vi "Update Sequence Params.vi"(8 "error in (no error)":errorcluster, 9 "Daq Channel Info In":T1, 10 "Sequence Parameters In":T2, 11 "UI in":refnum<class "UI.lvclass">) -> (0 "error out":errorcluster, 3 "UI out":refnum<class "UI.lvclass">)   [LabVIEW 2015, in "UI.lvlib" / "UI.lvclass"]
uses:
  UI.lvclass
  Sequencer/Sequencer/Sequence Parameters.ctl
  Sequencer/Sequencer/Daq Channel Info.ctl
  UI.lvclass/UI.ctl
  <vilib>/ActorFramework/Actor/Actor.lvclass/Actor.ctl
  <vilib>/ActorFramework/Message Enqueuer/Message Enqueuer.lvclass/Message Enqueuer.ctl
  <vilib>/ActorFramework/Message Enqueuer/Init from Existing Queue.vi
  <vilib>/ActorFramework/Message Enqueuer/Message Enqueuer.lvclass
  <vilib>/ActorFramework/Actor/Actor.lvclass
  UI Messages/Update Refs Msg/Update Refs Msg.lvclass
  Sequencer/Sequencer/Sequencer.lvclass
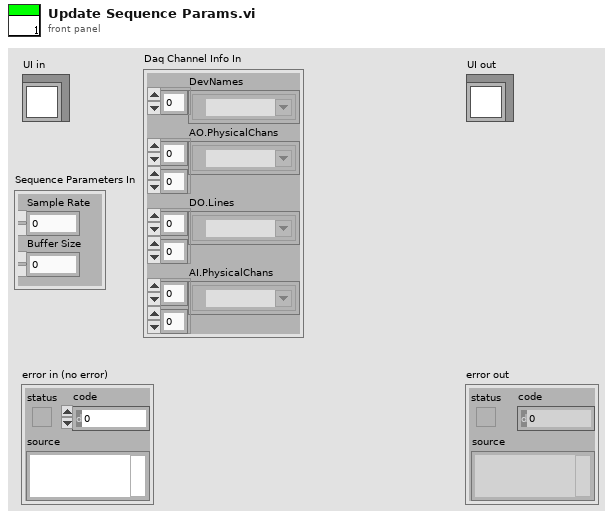
[diagram p1: front panel]
types:
  T1 = typedef "Sequencer.lvlib/Sequencer.lvclass/Daq Channel Info.ctl" = cluster{"DevNames":tag[], "AO.PhysicalChans":tag[][], "DO.Lines":tag[][], "AI.PhysicalChans":tag[][]}
  T2 = typedef "Sequencer.lvlib/Sequencer.lvclass/Sequence Parameters.ctl" = cluster{"Buffer Size":dbl, "Sample Rate":dbl}
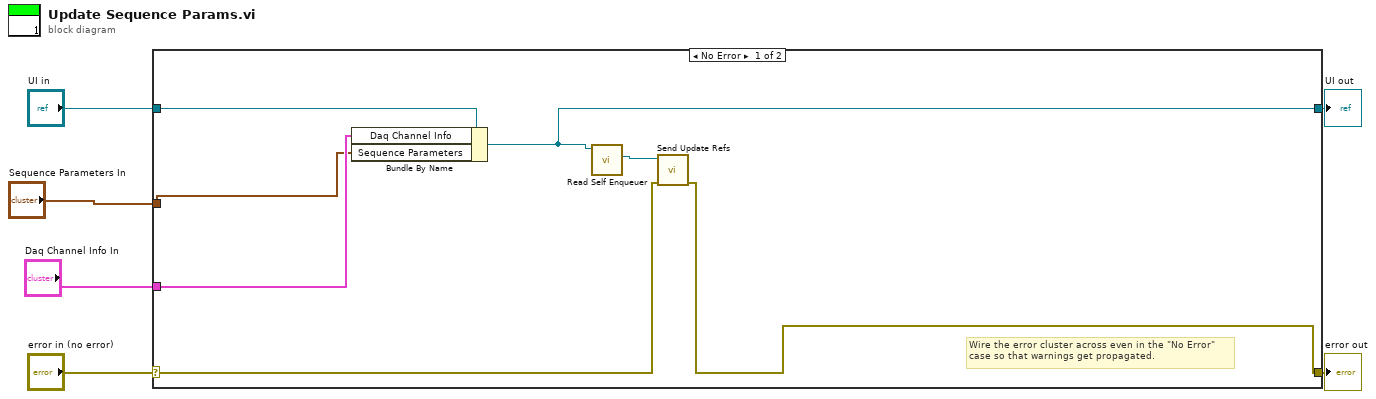
[diagram p0: block diagram]
diagram:
  n1 = case shown="No Error" "error in (no error)" {
    selector: "error in (no error)" -> [w9 w15]
    tunnel: [w7 w15] -> w5
    tunnel: [w8 w14] -> w3
    tunnel: "UI in" -> [w13 w14]
    tunnel: "Sequence Parameters In" -> [w11 _]
    tunnel: "Daq Channel Info In" -> [w12 _]
    frame No Error {
      # "Wire the error cluster across even in the \"No Error\"\ncase so that warnings get propagated."
      n2 = Bundle By Name(cluster=w13, "Daq Channel Info"=w12, "Sequence Parameters"=w11) -> (w8:refnum<class "UI.lvclass">)
      n3 = call <vilib>:"Read Self Enqueuer.vi"("Actor"=w8) -> ("Self Enqueuer"=w10:refnum<class "Message Enqueuer.lvclass">)  [unwired: 10 in]
      n4 = call "Send Update Refs.vi"("error in (no error)"=w9, "Message Enqueuer in"=w10) -> ("error out"=w7:errorcluster)  [unwired: 8 in, 1 out]
    }
    frame Error {
    }
  }
  "error out" <- w5
  "UI out" <- w3
